vi "rad_Apply Network Settings (DHCP).vi"(5 "Password":string, 8 "error in (no error)":errorcluster, 10 "Requested settings":T1={"Hostname"="", "Serial number"="", "Product name"="", "Product code"=0, "System status"="", "Credential type"=enum."None/Unlocked", "User added?"=FALSE, "Primary NIC"={"MAC address"="", "IP Address Request Mode"=2, "IP address"="", "Subnet mask"="", "Gateway"="", "DNS server"=""}} {"Primary NIC"."IP Address Request Mode" items=["Static"=1, "DHCP/Link-Local"=2, "Link-Local Only"=4, "DHCP Only"=8]}, 11 "Existing settings":T1={"Hostname"="", "Serial number"="", "Product name"="", "Product code"=0, "System status"="", "Credential type"=enum."None/Unlocked", "User added?"=FALSE, "Primary NIC"={"MAC address"="", "IP Address Request Mode"=2, "IP address"="", "Subnet mask"="", "Gateway"="", "DNS server"=""}} {"Primary NIC"."IP Address Request Mode" items=["Static"=1, "DHCP/Link-Local"=2, "Link-Local Only"=4, "DHCP Only"=8]}) -> (0 "error out":errorcluster, 3 "Target settings out":T1={"Hostname"="", "Serial number"="", "Product name"="", "Product code"=0, "System status"="", "Credential type"=enum."None/Unlocked", "User added?"=FALSE, "Primary NIC"={"MAC address"="", "IP Address Request Mode"=2, "IP address"="", "Subnet mask"="", "Gateway"="", "DNS server"=""}} {"Primary NIC"."IP Address Request Mode" items=["Static"=1, "DHCP/Link-Local"=2, "Link-Local Only"=4, "DHCP Only"=8]})   [LabVIEW 2020]
uses:
  <vilib>/nisyscfg/nisyscfg.lvlib
  <resource>/objmgr/nisysapi.rc
  <vilib>/nisyscfg/Save Changes (System).vi
  <vilib>/nisyscfg/Close (System).vi
  rad_Globals.vi
  TypeDefs/rad_Target Information.ctl
  TypeDefs/rad_Target Network Settings.ctl
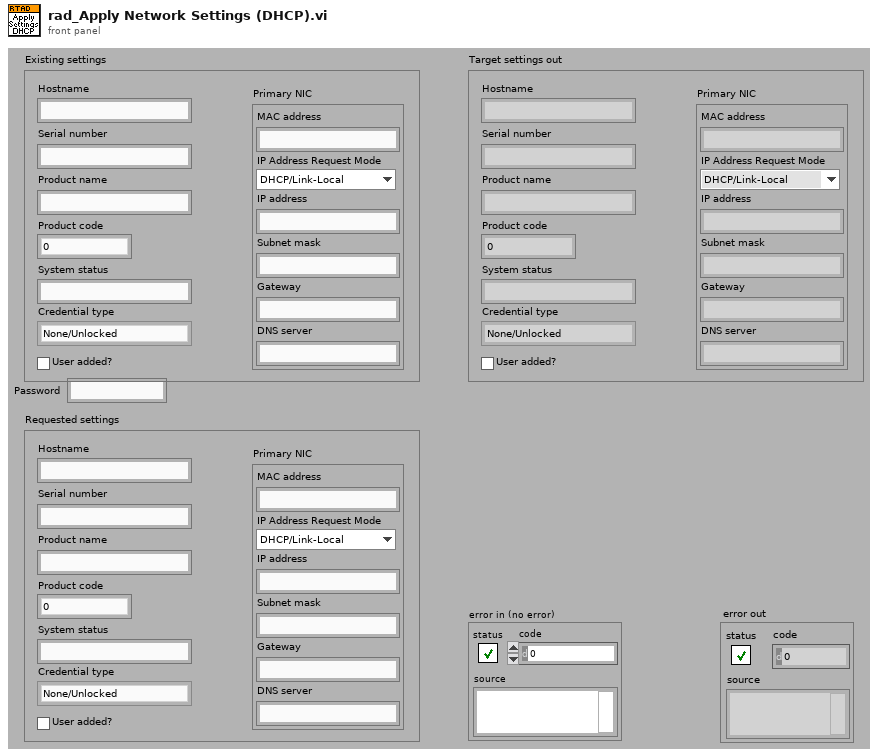
[diagram p1: front panel]
types:
  T1 = typedef "rad_Target Information.ctl" = cluster{"Hostname":string, "Serial number":string, "Product name":string, "Product code":i32, "System status":string, "Credential type":enum16{"None/Unlocked", "FTP Password", "NIAuth Credentials"}, "User added?":bool, "Primary NIC":T2}
  T2 = typedef "rad_Target Network Settings.ctl" = cluster{"MAC address":string, "IP Address Request Mode":i32, "IP address":string, "Subnet mask":string, "Gateway":string, "DNS server":string}
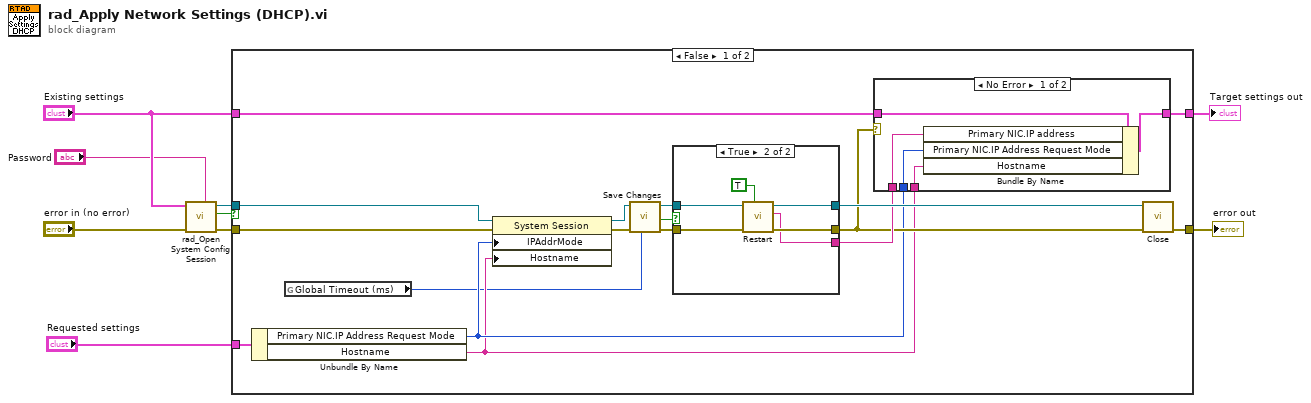
[diagram p0: block diagram]
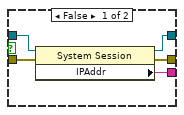
[diagram p3: hidden frame]
diagram:
  n1 = call "rad_Open System Config Session.vi"("Password"="Password", "error in (no error)"="error in (no error)", "Target settings"="Existing settings") -> ("error out"=w6:errorcluster, "Cancelled"=w5:bool, "Session out"=w7:refnum<k21>)  [unwired: 5 in, 1 out]
  n2 = case shown="False" w5 {
    tunnel: w7 -> [w26 _]
    tunnel: w6 -> [w25 w45]
    tunnel: [w24 w45] -> w8
    tunnel: "Existing settings" -> [w18 w44]
    tunnel: [w17 w44] -> w4
    tunnel: "Requested settings" -> [w13 _]
    frame False {
      n3 = Unbundle By Name(w13) -> ("Primary NIC.IP Address Request Mode"=w12:i32, "Hostname"=w11:string)
      n4 = global read "rad_Globals.vi" "Global Timeout (ms)"() -> (w10:u32)
      n5 = property class="System Session"(reference=w26, error in=w25, "IPAddrMode"=w12, "Hostname"=w11) -> (reference out=w23:refnum<k21>, error out=w22:errorcluster)
      n6 = call-poly <vilib>:"Save Changes.vi"("Remote Timeout (300,000 ms)"=w10, "error in (no error)"=w22, "Session in"=w23) -> ("error out"=w20:errorcluster, "Changes Require Restart"=w21:bool, "Session out"=w19:refnum<k21>)  [unwired: 5 in, 1 out]
      n7 = case shown="True" w21 {
        tunnel: w20 -> [w37 w43]
        tunnel: [w36 w42] -> w14
        tunnel: w19 -> [w35 w41]
        tunnel: [w34 w40] -> w16
        tunnel: [w33 w38] -> w15
        frame False {
          n8 = property class="System Session"(reference=w35, error in=w37) -> (reference out=w34:refnum<k21>, error out=w36:errorcluster, "IPAddr"=w33:string)
        }
        frame True {
          n9 = call <vilib>:"Restart.vi"("Wait Until Complete (T)"=TRUE ("wait until complete (T)"), "error in (no error)"=w43, "Session in"=w41) -> ("error out"=w42:errorcluster, "New IP Address"=w38:string, "Session out"=w40:refnum<k21>)  [unwired: 6 in]
        }
      }
      n10 = case shown="No Error" w14 {
        tunnel: w18 -> [w31 w32]
        tunnel: [w30 w32] -> w17
        tunnel: w11 -> [w29 _]
        tunnel: w12 -> [w28 _]
        tunnel: w15 -> [w27 _]
        frame No Error {
          n11 = Bundle By Name(cluster=w31, "Primary NIC.IP address"=w27, "Primary NIC.IP Address Request Mode"=w28, "Hostname"=w29) -> (w30:T1)
        }
        frame Error {
        }
      }
      n12 = call-poly <vilib>:"Close.vi"("error in (no error)"=w14, "Session in"=w16) -> ("error out"=w24:errorcluster)  [unwired: 9 in]
    }
    frame True {
    }
  }
  "error out" <- w8
  "Target settings out" <- w4
